vi "Select Channel Dialog.vi"(8 "error in (no error)":errorcluster, 11 "NIVS.System Definition Root":refnum<k24>) -> (0 "error out":errorcluster, 2 "Cancel?":bool, 3 "Selected Item":T1)   [LabVIEW 2023, in "J1939 Workspace Shared.lvlib"]
uses:
  J1939 Workspace Shared.lvlib
  NationalInstruments.VeriStand.SystemStorageUI
  NationalInstruments.VeriStand.SystemStorage
  <vilib>/NI VeriStand/UI Controls/Single Node Browser/Node Ref.ctl
  <vilib>/NI VeriStand/UI Controls/Single Node Browser/NI_VS UI Single Node Browser.lvlib
panel:
  in  "Single Node Browser":refnum<k24>(container)
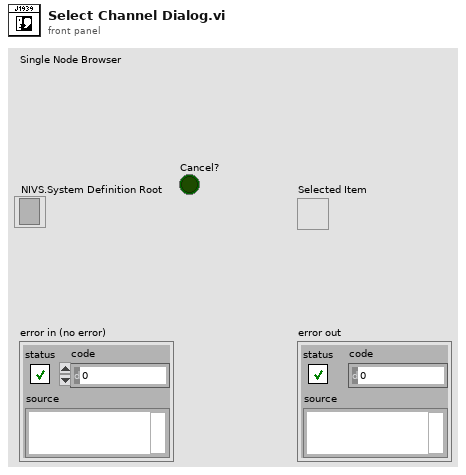
[diagram p1: front panel]
types:
  T1 = typedef "NI_VS UI Single Node Browser.lvlib/Node Ref.ctl" = refnum<k24>
  T2 = typedef "NI_VS UI Single Node Browser.lvlib/Callback Type.ctl" = cluster{"Net Callbacks":refnum<k27>[], "Event":refnum<user-event>}
  T3 = typedef "NI_VS UI Single Node Browser.lvlib/Single Node Browser Ref.ctl" = refnum<k24>
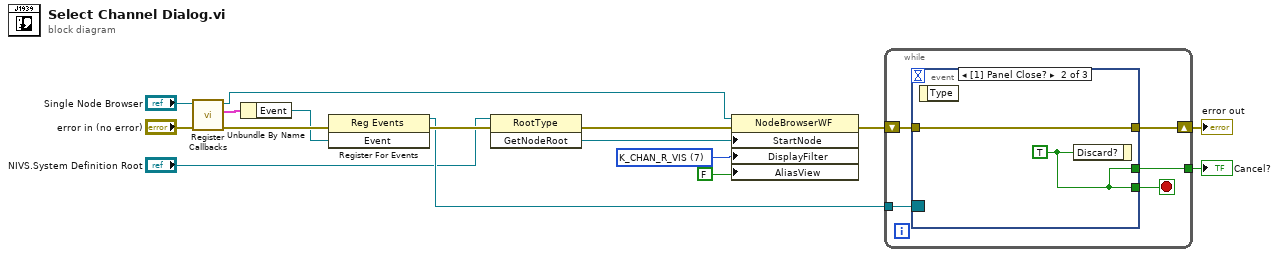
[diagram p0: block diagram]
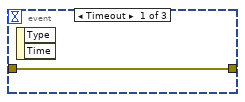
[diagram p2: hidden frame]
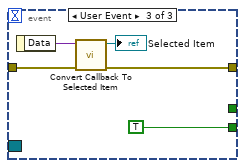
[diagram p3: hidden frame]
diagram:
  w11 = u8 7 items=["K_CHAN_R", "K_CHAN_W", "K_CHAN_RW", "K_CHAN_VOLT", "K_CHAN_FAULT", "K_ALL", "K_CUSTOM", "K_CHAN_R_VIS", "K_CHAN_W_VIS", "K_CHAN_RW_VIS", "K_CHAN_VOLT_VIS", "K_CHAN_FAULT_VIS"] ("DisplayFilter")
  n1 = call <vilib>:"Register Callbacks.vi"("error in (no error)"="error in (no error)", "Single Node Browser"="Single Node Browser") -> ("error out"=w14:errorcluster, "Callbacks"=w15:T2, "Single Node Browser dup"=w8:T3)  [unwired: 7 in]
  n2 = Unbundle By Name(w15) -> ("Event"=w13:refnum<user-event>)
  n3 = register-events(error in=w14, w13) -> (reference out=w6:refnum<event-registration>, error out=w9:errorcluster)  [unwired: 1 in]
  n4 = invoke class="RootType" method="GetNodeRoot"(reference="NIVS.System Definition Root", error in=w9) -> (error out=w16:errorcluster, "GetNodeRoot"=w10:refnum<k24>)  [unwired: 1 in, 1 out]
  n5 = property class="NodeBrowserWF"(reference=w8, error in=w16, "StartNode"=w10, "DisplayFilter"=w11, "AliasView"=FALSE) -> (error out=w5:errorcluster)  [unwired: 1 out]
  n6 = while {
    tunnel: w6 -> [w21]
    shift-right: [w19] -> w4
    shift-left: w5 -> [w18]
    tunnel: [w17] -> w2
    stop <- w20 stop-if-true
    n7 = event shown="[1] Panel Close?" {
      selector: w21 -> [_ _ _]
      dyn-events: _ -> [_ _ _]
      timeout: _ -> [_ _ _]
      tunnel: [_ w23 TRUE] -> w20
      tunnel: w18 -> [w22 w24 w26]
      tunnel: [w22 w24 w25] -> w19
      tunnel: [_ w23 _] -> w17
      event Timeout {
        n8 = event-data() -> ()  [unwired: 1 in, 2 out]
      }
      event Panel Close? {
        w23 = TRUE ("Discard?")
        n9 = event-data() -> ()  [unwired: 1 in, 1 out]
        n10 = event-data("Discard?"=w23) -> ()  [unwired: 1 in, 1 out]
      }
      event User Event {
        n11 = event-data() -> ("Data"=w29:variant)  [unwired: 1 in]
        n12 = call <vilib>:"Convert Callback To Selected Item.vi"("error in"=w26, "Data"=w29) -> ("error out"=w25:errorcluster, "Selected Item"=→"Selected Item":T1)  [unwired: 8 in]
      }
    }
  }
  "error out" <- w4
  "Cancel?" <- w2
